vi "OCR_Build Bit array.vi"(7 "Color Set":T2, 8 "Error":errorcluster, 9 "Index":i16, 10 "Width":i32, 11 "2D Image":u32[][](array[colorbox])) -> (0 "Error Out":errorcluster, 3 "Bit Array Out":T1)   [LabVIEW 2009]
doc: "Builds a character bit array from the index width and color set"
uses:
  Controls/Cluster/Cluster_Text Color Set.ctl
  Controls/Array/Array Bool Char Bits Wide.ctl
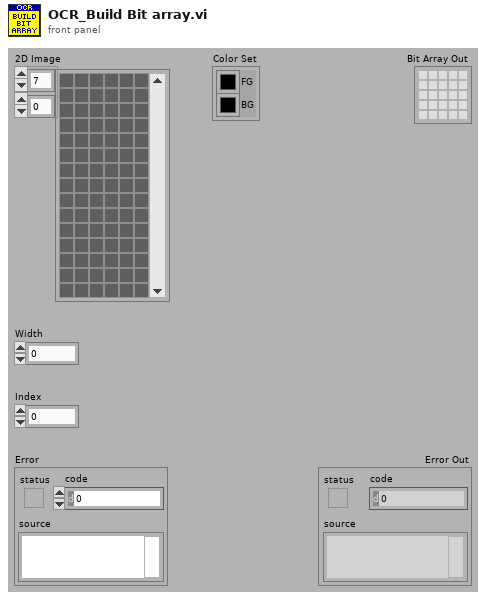
[diagram p1: front panel]
types:
  T1 = typedef "Array Bool Char Bits Wide.ctl" = bool[][]
  T2 = typedef "Cluster_Text Color Set.ctl" = cluster{"BG":u32, "FG":u32}
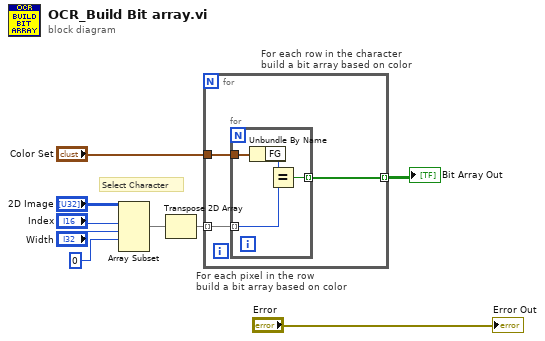
[diagram p0: block diagram]
diagram:
  # "Select Character"
  n1 = Array Subset(array="2D Image", index (row)="Index", length (row)="Width", index (col)=0 ("index")) -> (w6:u32[][])  [unwired: 1 in]
  n2 = Transpose 2D Array(2D array=w6) -> (transposed array=w7:u32[][])
  n3 = for "For each row in the character\nbuild a bit array based on color" {
    tunnel: w7 -> [w12] mode=indexing
    tunnel: "Color Set" -> [w11]
    tunnel: [w10] -> w2 mode=indexing
    n4 = for "For each pixel in the row\nbuild a bit array based on color" {
      tunnel: w12 -> [w14] mode=indexing
      tunnel: w11 -> [w16]
      tunnel: [w13] -> w10 mode=indexing
      n5 = Unbundle By Name(w16) -> ("FG"=w15:u32)
      n6 = Equal?(x=w15, y=w14) -> (x = y?=w13:bool)
    }
  }
  "Bit Array Out" <- w2
  "Error Out" <- "Error"
